vi "整体正交拟合.vi"() -> ()   [LabVIEW 2014]
uses:
  <vilib>/Analysis/NI_AALBase.lvlib
  <vilib>/Analysis/baseanly.llb/Normalize Vector.vi
panel:
  in  "添加的数组":cluster{"Array":dbl[], "Array":dbl[]}[](array[cluster])
  in  "拟合阶次":i32
  in  "迭代次数":i32
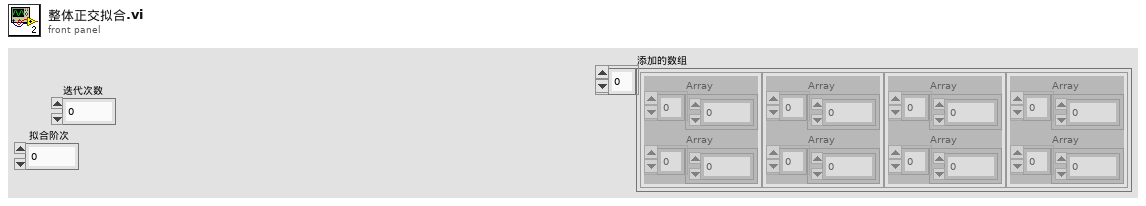
[diagram p1: front panel]
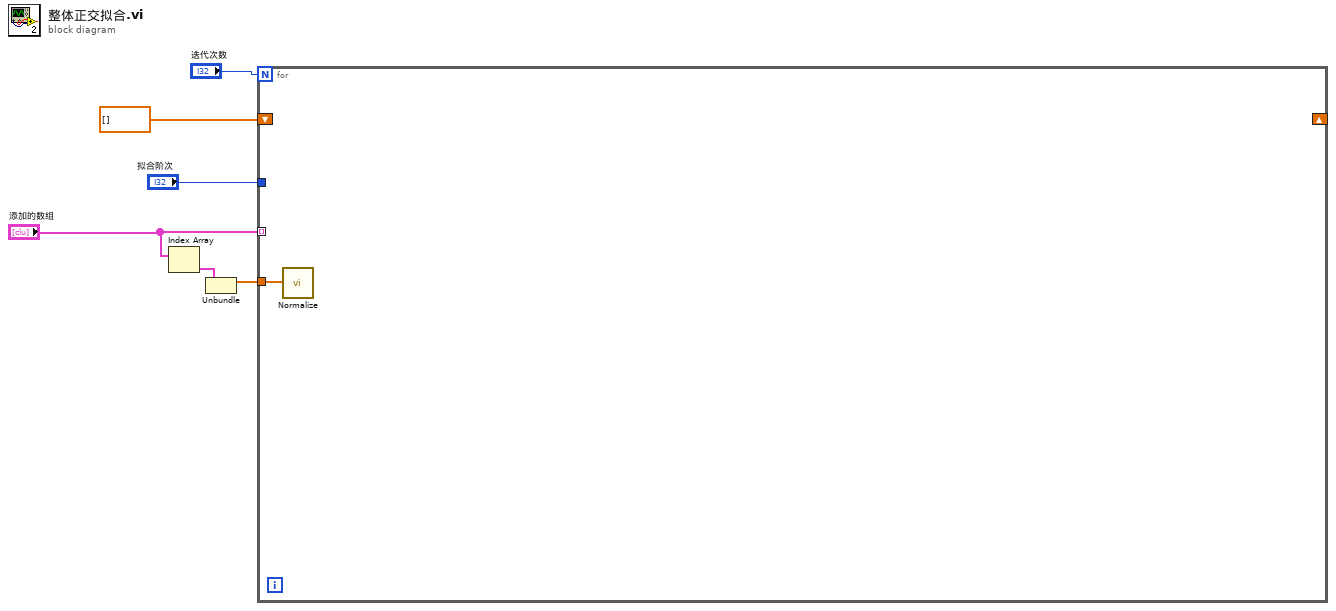
[diagram p0: block diagram]
diagram:
  n1 = Index Array(array="添加的数组") -> (element=w3:cluster{"Array":dbl[], "Array":dbl[]})  [unwired: 1 in]
  n2 = Unbundle(w3) -> ("Array"=w1:dbl[])  [unwired: 1 out]
  n3 = for {
    N: "迭代次数" -> [_]
    shift-right: _ -> [_]
    shift-left: dbl[] [] -> [_]
    tunnel: "拟合阶次" -> [_]
    tunnel: [w8] -> _
    tunnel: "添加的数组" -> [w8] mode=indexing
    tunnel: w1 -> [w7]
    n4 = call-poly <vilib>:"Normalize.vi"("Vector"=w7) -> ()  [unwired: 1 in, 4 out]
  }
